vi "PS_ReadVolt_Current.vi"(8 "error in (no error)":errorcluster, 11 "VISA resource name":refnum<visa-resource-name>) -> (0 "error out":errorcluster, 2 "Current":dbl, 3 "Volt":dbl)   [LabVIEW 2018, in "Acquire Data.lvclass"]
uses:
  Acquire Data.lvclass
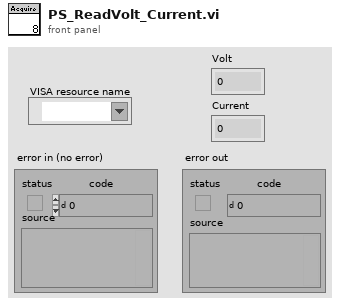
[diagram p1: front panel]
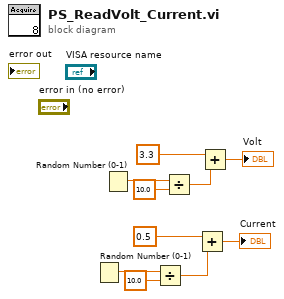
[diagram p0: block diagram]
diagram:
  n1 = Random Number (0-1)() -> (number: 0 to 1=w4:dbl)
  n2 = Random Number (0-1)() -> (number: 0 to 1=w10:dbl)
  n3 = Divide(x=w4, y=10.0) -> (x/y=w3:dbl)
  n4 = Divide(x=w10, y=10.0) -> (x/y=w7:dbl)
  n5 = Add(x=0.5, y=w3) -> (x+y=→"Current":dbl)
  n6 = Add(x=3.3, y=w7) -> (x+y=→"Volt":dbl)
